vi "Configure DO Fail.vi"(0 "VISA resource name":refnum<visa-resource-name>, 5 "Channel Number (0001)":string="0001", 7 "Span And Energize":T1={"Span Lower Limit (0)"=0, "Span Upper Limit (1)"=1, "Unit (\"\")"=""} {"Span Upper Limit (1)" min=1 max=32; "Span Lower Limit (0)" min=1 max=32}, 11 "error in (no error)":errorcluster) -> (4 "VISA resource name out":refnum<visa-resource-name>, 6 "Channel Number":string, 15 "error out":errorcluster)   [LabVIEW 2020, in "Yokogawa GX Series.lvlib"]
doc: "Sets the DO fail output related settings.\n\nCommand: SRangeDO"
uses:
  <instrlib>/Yokogawa GX Series/Yokogawa GX Series.lvlib
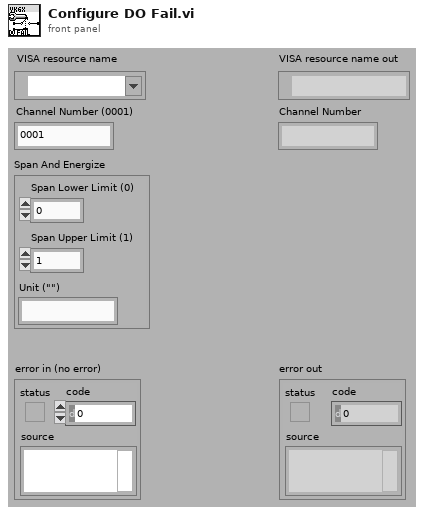
[diagram p1: front panel]
types:
  T1 = cluster{"Span Lower Limit (0)":i32, "Span Upper Limit (1)":i32, "Unit (\"\")":string}
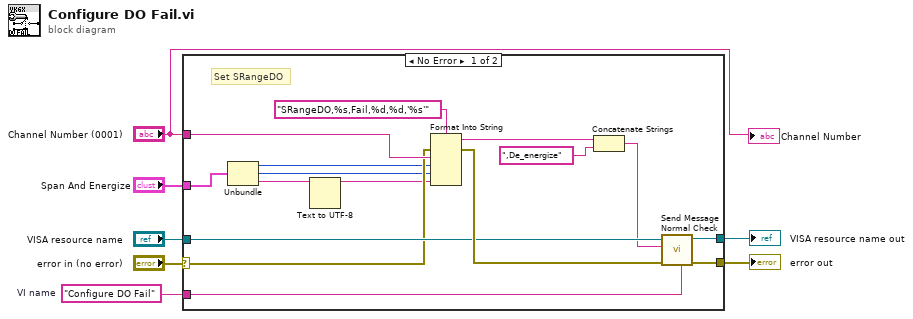
[diagram p0: block diagram]
diagram:
  w7 = "Configure DO Fail"  # VI name
  n1 = case shown="No Error" "error in (no error)" {
    selector: "error in (no error)" -> [w16 w24]
    tunnel: w7 -> [w23 _]
    tunnel: [w22 w25] -> w6
    tunnel: [w21 w24] -> w5
    tunnel: "VISA resource name" -> [w18 w25]
    tunnel: "Span And Energize" -> [w15 _]
    tunnel: "Channel Number (0001)" -> [w17 _]
    frame No Error {
      # "Set SRangeDO"
      n2 = Unbundle(w15) -> ("Span Lower Limit (0)"=w14:i32, "Span Upper Limit (1)"=w13:i32, "Unit (\"\")"=w9:string)
      n3 = Text to UTF-8(11:w9) -> (3:w8:string)  [unwired: 2 in, 1 out]
      n4 = Format Into String(format string="SRangeDO,%s,Fail,%d,%d,'%s'" ("形式文字列"), error in=w16, w17, w14, w13, w8) -> (resulting string=w12:string, error out=w19:errorcluster)  [unwired: 1 in]
      n5 = Concatenate Strings(w12, ",De_energize") -> (w10:string)
      n6 = call <instrlib>:"Send Message Normal Check.vi"("Source (\"\")"=w23, "error in (no error)"=w19, "Send Message (\"\")"=w10, "VISA resource name"=w18) -> ("error out"=w21:errorcluster, "VISA resource name out"=w22:refnum<visa-resource-name>)  [unwired: 1 in, 5 out]
    }
    frame Error {
    }
  }
  "error out" <- w5
  "VISA resource name out" <- w6
  "Channel Number" <- "Channel Number (0001)"
